vi "Main.vi"() -> ()   [LabVIEW 2012]
uses:
  <vilib>/addons/_XControls/Orbit Plot/SVX Orbit.xctl
  <vilib>/Math Plots/3D Math Plots/3D Surface/3D Surface XCtrl/3D Surface.xctl
  <vilib>/Utility/error.llb/DialogType.ctl
  <vilib>/Analysis/3filter.llb/Filter Passband Type.ctl
  <vilib>/DAQmx/read.llb/DAQmx Read (Analog 1D Wfm NChan NSamp).vi
  <vilib>/DAQmx/create/channels.llb/DAQmx Create Channel (AI-Position-EddyCurrentProxProbe).vi
  <vilib>/DAQmx/configure/timing.llb/DAQmx Timing (Sample Clock).vi
  <vilib>/Waveform/WDTOps.llb/WDT Append Waveforms DBL.vi
  <vilib>/Waveform/WDTOps.llb/WDT Index Channel DBL.vi
  <vilib>/Analysis/baseanly.llb/Mean (DBL).vi
  <vilib>/Waveform/WDTOps.llb/WDT Index Channel by Name DBL.vi
  <vilib>/Analysis/3filter.llb/Butterworth Filter (DBL).vi
  <vilib>/DAQmx/miscellaneous.llb/DAQmx Fill In Error Info.vi
  <resource>/objmgr/daqmx.rc
  <vilib>/Analysis/NI_AALBase.lvlib
  <vilib>/addons/Sound and Vibration/Order Analysis/Tach Process/SoundVib_TachProcess.lvlib
panel:
  out "3D Surface":refnum<class "3D Plot Datatype.lvclass">[](xcontrol)
  out "owmax":dbl
  out "Oil Whirl":T1(graph)
  out "Freq [Hz]":dbl
  out "deltaphase":dbl
  out "even-angle references":cluster{"r0":dbl, "dr":dbl, "Y":dbl[]}[](array[cluster])
  out "Magcri2":dbl
  out "Freq [Hz]":dbl
  out "Partial Rub":T1(graph)
  out "Freq [Hz]":dbl
  out "MATSCRIPT error 3":errorcluster
  out "prmax":dbl
  out "FreqFspec":T2(array[cluster])
  out "Freq [Hz]":dbl
  out "Unbalance":T1(graph)
  out "Freq crit":dbl
  out "Magcrit":dbl
  out "Radial Load/ Rotor cracked":T1(graph)
  out "RotMagdeltaphase":dbl[](array[numeric])
  out "MATSCRIPT error 2":errorcluster
  out "Full Spectro error":errorcluster
  out "error dequeue 2":errorcluster caption="error out"
  out "# elements in queue FS":i32
  out "> Limit":bool
  out "Actual Sample Rate (dt)":dbl
  out "MATSCRIPT error":errorcluster
  out "RPMs Calculados":i32
  out "Channels and Names":string[][](array[string])
  in  "Start":bool
  out "State":T3(ring)
  out "error dequeue":errorcluster caption="error out"
  out "Mag/F":errorcluster
  out "no tacho?":bool
  out "# elements in queue":i32
  out "> limit":bool
  in  "Stop":bool
  in  "Tab Control":T4(tab)
  in  "Names":string[](array[string])
  in  "Min Sample Rate [Hz]":dbl=10000.0
  in  "Maximum Value":dbl=0.0025 format="%.5f"
  in  "Units":i32(ring)=10219 items=["Meters"=10219, "Inches"=10379, "From Custom Scale"=10065]
  in  "Sensitivity":dbl=7.87
  in  "Sensitivity Units":i32(ring)=14839 items=["mVolts/mil"=14836, "Volts/mil"=14837, "mVolts/mm"=14838, "Volts/mm"=14839, "mVolts/micron"=14840]
  in  "Minimum Value":dbl=0.0002 format="%.5f"
  in  "DAQmx Selector":cluster{"On":bool, "physical channels":tag}[](array[cluster])=[{"On"=TRUE, "physical channels"="cDAQ2Mod1/ai0"}, {"On"=TRUE, "physical channels"="cDAQ2Mod1/ai1"}, {"On"=TRUE, "physical channels"="cDAQ2Mod1/ai2"}, {"On"=TRUE, "physical channels"="cDAQ2Mod2/ai0"}]
  in  "Keyphasor":tag="cDAQ2Mod2/ai1"
  in  "Threshold":dbl=0.0001
  in  "Direction":enum16{"CCW", "CW"}(ring)
  out "Actual Sample Rate [Hz]":dbl
  in  "Probe Angle X [deg]":u16
  in  "Probe Angle Y [deg]":u16=90
  out "Keyphasor":waveform(dbl)(graph)
  out "Radial Sensors":waveform(dbl)[](graph)
  in  "Write to File?":bool
  in  "TDMS File Path":path=path "C:/Users/Clayton/Documents/Mestrado ITA/Dissertacao/Simulacoes Matlab/zLabView/TDMS_teste.tdms"
  in  "Axis Y - Orbit 2":i8(ring) items=["x1", "y1", "x2", "y2"]
  in  "Axis X - Orbit 1":i8(ring) items=["x1", "y1", "x2", "y2"]
  out "Orbit 1":cluster{"Y":dbl[], "Y":dbl[]}(graph)
  out "Orbit 2":cluster{"Y":dbl[], "Y":dbl[]}(graph)
  in  "Axis Y - Orbit 1":i8(ring) items=["x1", "y1", "x2", "y2"]
  in  "Axis X - Orbit 2":i8(ring) items=["x1", "y1", "x2", "y2"]
  in  "Automatic":dbl=10.0
  in  "Duration [Rotation]":dbl=10.0 format="%.2f"
  in  "Sensor Y":i8(ring) items=["x1", "y1", "x2", "y2"]
  in  "Sensor X":i8(ring) items=["x1", "y1", "x2", "y2"]
  out "Full Spectrum":T1(graph)
  in  "Window":u32(ring)=1 items=["None"=0, "Hanning"=1, "Hamming"=2, "Blackman-Harris"=3, "Exact Blackman"=4, "Blackman"=5, "Flat Top"=6, "4 Term B-Harris"=7, "7 Term B-Harris"=8, "Low Sidelobe"=9, "Gaussian"=62]
  out "Rotor Crack":dbl(slide) scale=0.0..1.0
  out "Partial Rub":dbl(slide) scale=0.0..1.0
  out "Radial Load":dbl(slide) scale=0.0..1.0
  out "Unbalance":dbl(slide) scale=0.0..1.0
  out "Oil Whirl":dbl(slide) scale=0.0..1.0
  out "Rotation [rps]":dbl format="%#.4f"
  out "Error Matlab Script":bool
  out "Error Full Spectrum":bool
  in  "Compensate":bool
  in  "Reset":bool
  out "Orbit Plot":T5(xcontrol)
  in  "Freq. Diagnosis [rps]":dbl=50.0
  in  "Simulation path":path=path "C:/Users/Clayton/Documents/Mestrado ITA/Dissertacao/Simulacoes Matlab/zLabView/TDMS_teste.tdms"
  in  "Simulation":bool
  in  "Sensor X":i32=1
  in  "Sensor Y":i32=2
  out "Phase":cluster{dbl[], dbl[]}(graph)
  in  "Order":i8(ring) items=["1x", "2x"]
  out "Magnitude":cluster{dbl[], dbl[]}(graph)
  out "Phase":cluster{dbl[], dbl[]}(graph)
  out "Magnitude":cluster{dbl[], dbl[]}(graph)
  in  "Order":i8(ring) items=["1x", "2x"]
  out "Sensor":string
  out "Sensor":string
  # "Slow Roll"
  # "Diagnosis"
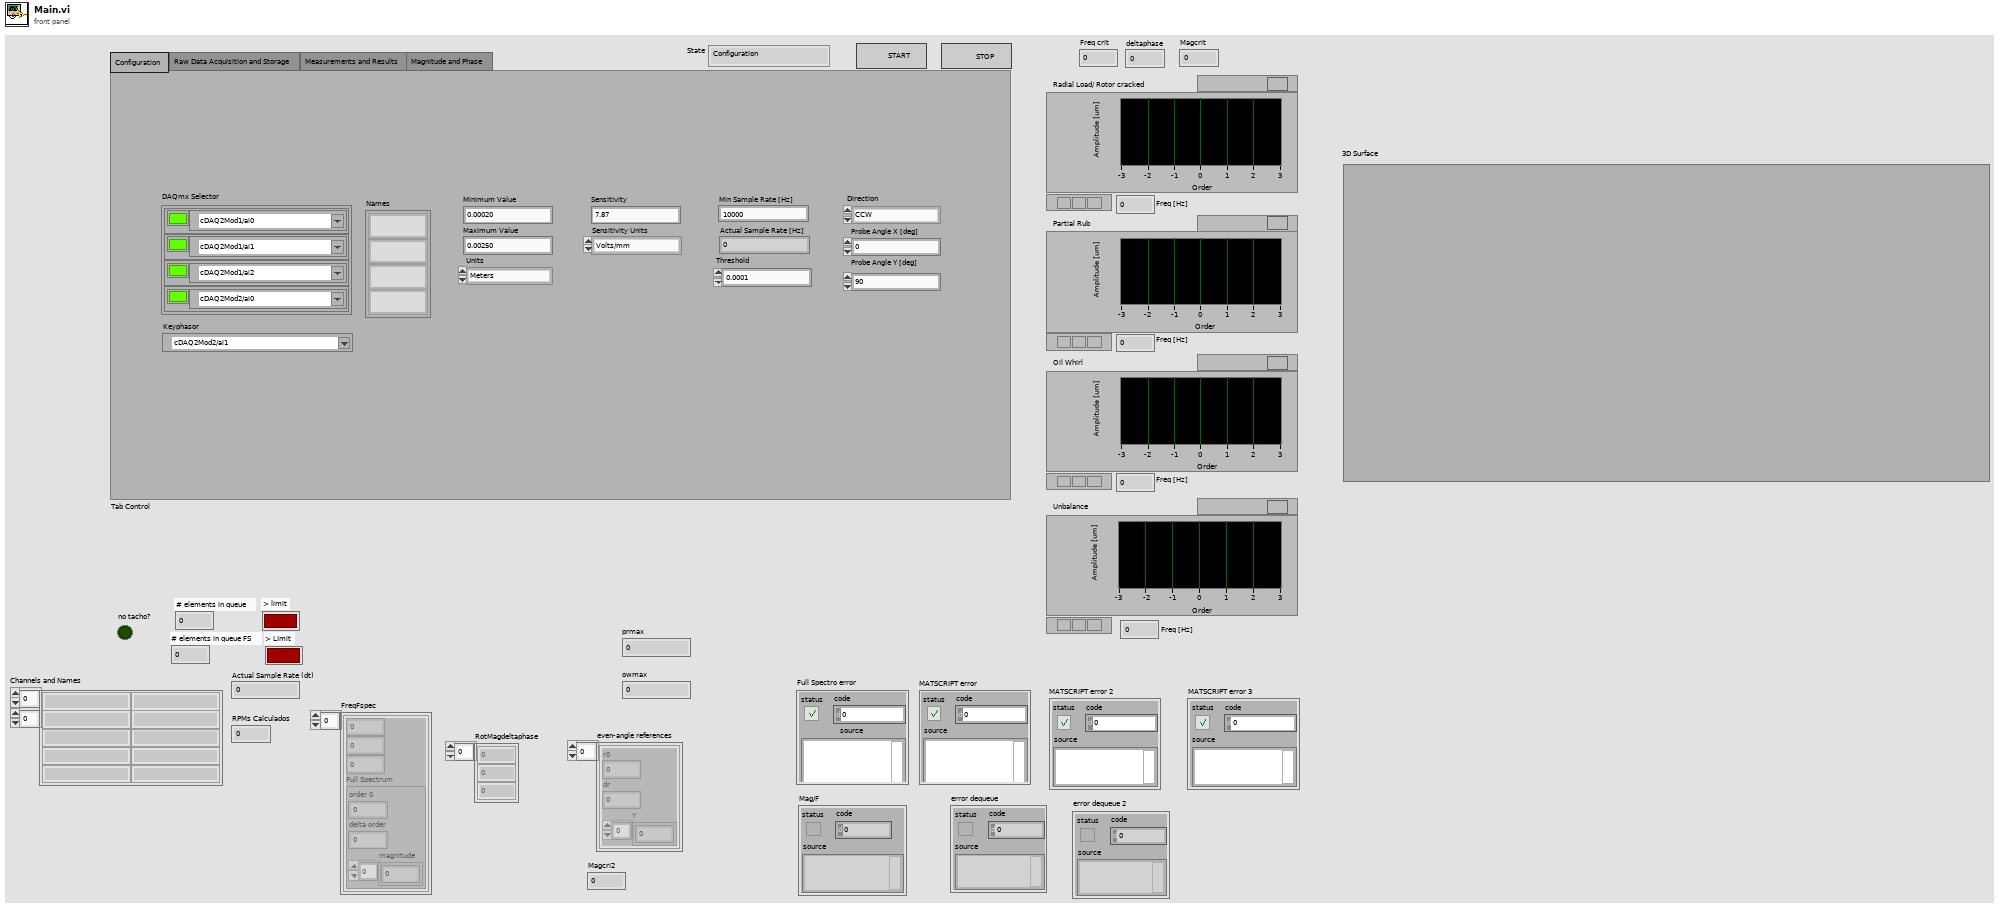
[diagram p1: front panel]
types:
  T1 = cluster{"order 0":dbl, "delta order":dbl, "magnitude":dbl[]}
  T2 = cluster{dbl, dbl, dbl, "Full Spectrum":cluster{"order 0":dbl, "delta order":dbl, "magnitude":dbl[]}}[]
  T3 = enum16{"Configuration", "Initializing", "RUNNING"}
  T4 = enum32{"Configuration", "Raw Data Acquisition and Storage", "Measurements and Results", "Magnitude and Phase"}
  T5 = cluster{"probe x":dbl[], "probe y":dbl[], "reference":dbl[], "plot type":enum16{"Filtered Plot", "Unfiltered Plot"}, "attribute":variant}[][]
  T6 = enum8{"Enabled", "Disabled", "Disabled and Grayed Out"}
  T7 = enum16{"open", "open or create", "create or replace", "create", "open (read-only)"}
  T8 = cluster{"dB on? (F)":bool, "unwrap phase? (T)":bool, "unit in degree? (T)":bool}
  T9 = typedef "DialogType.ctl" = u16
  T10 = typedef "NI_AALBase.lvlib/Filter Passband Type.ctl" = enum32{"Lowpass", "Highpass", "Bandpass", "Bandstop"}
  T11 = cluster{dbl, dbl, dbl, "Full Spectrum":cluster{"order 0":dbl, "delta order":dbl, "magnitude":dbl[]}}
  T12 = typedef "SoundVib_TachProcess.lvlib/speed profile.ctl" = cluster{"time [s]":dbl[], "speed [RPM]":dbl[]}
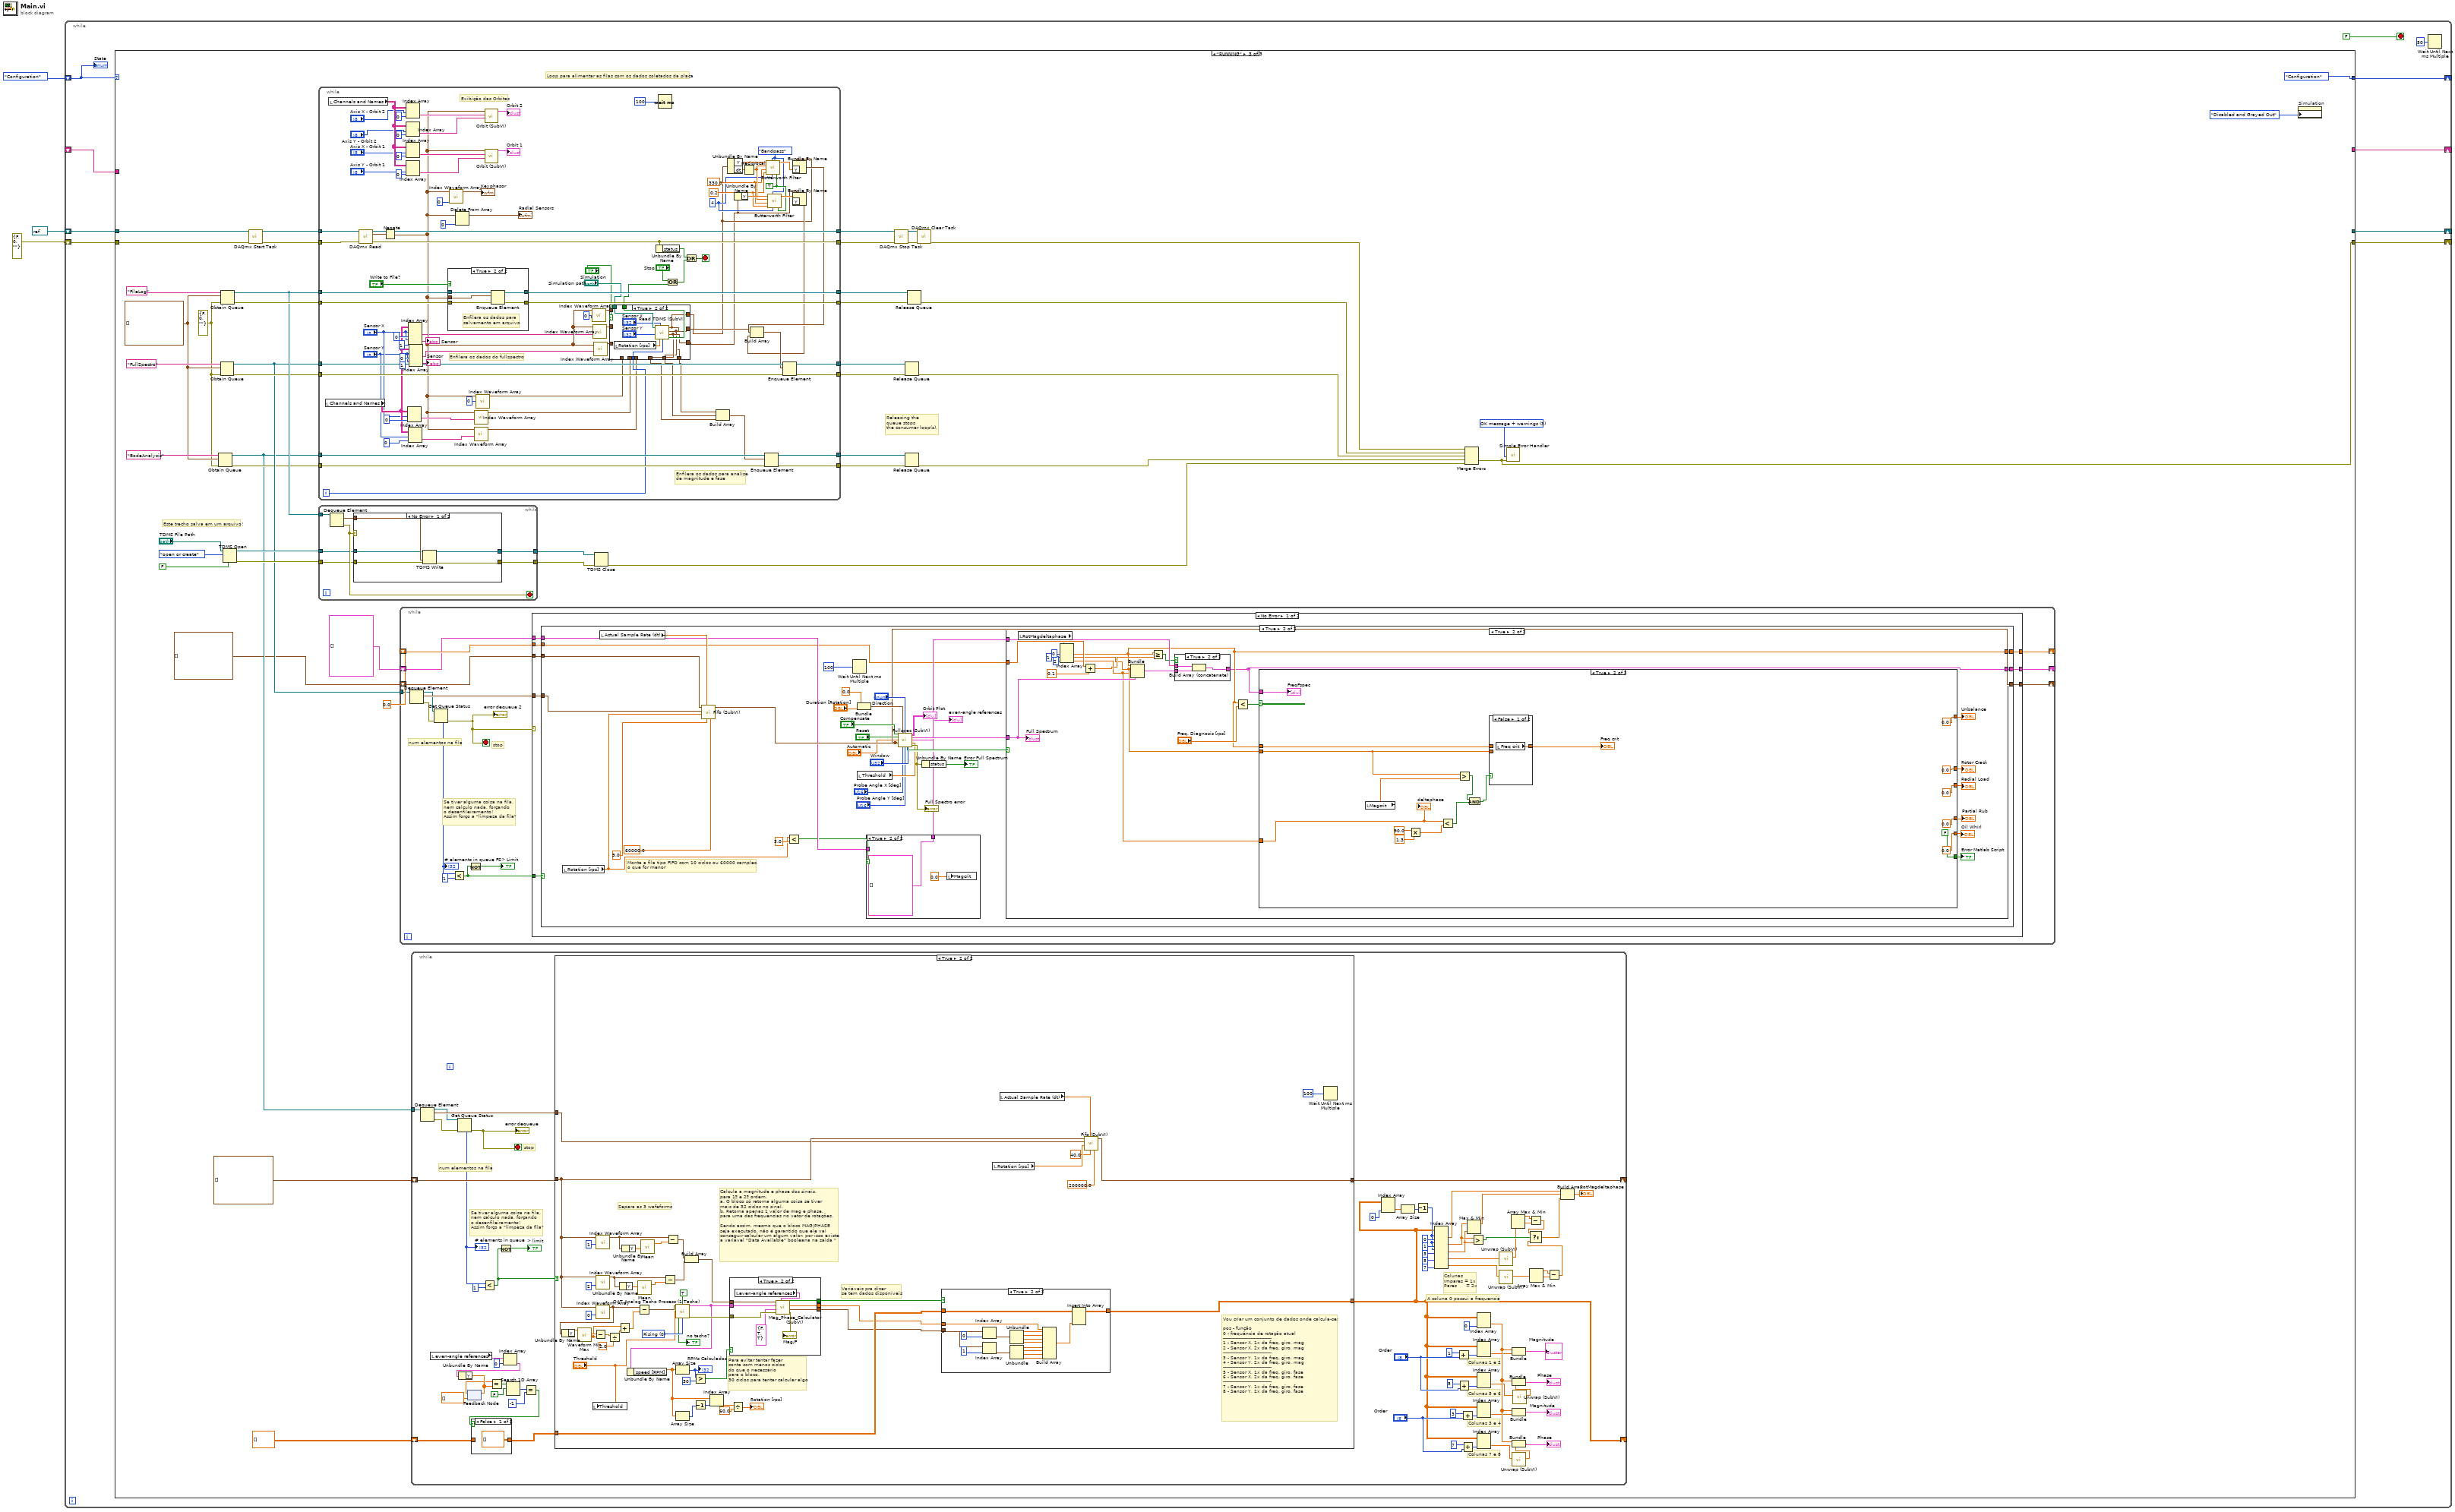
[diagram p0: block diagram]
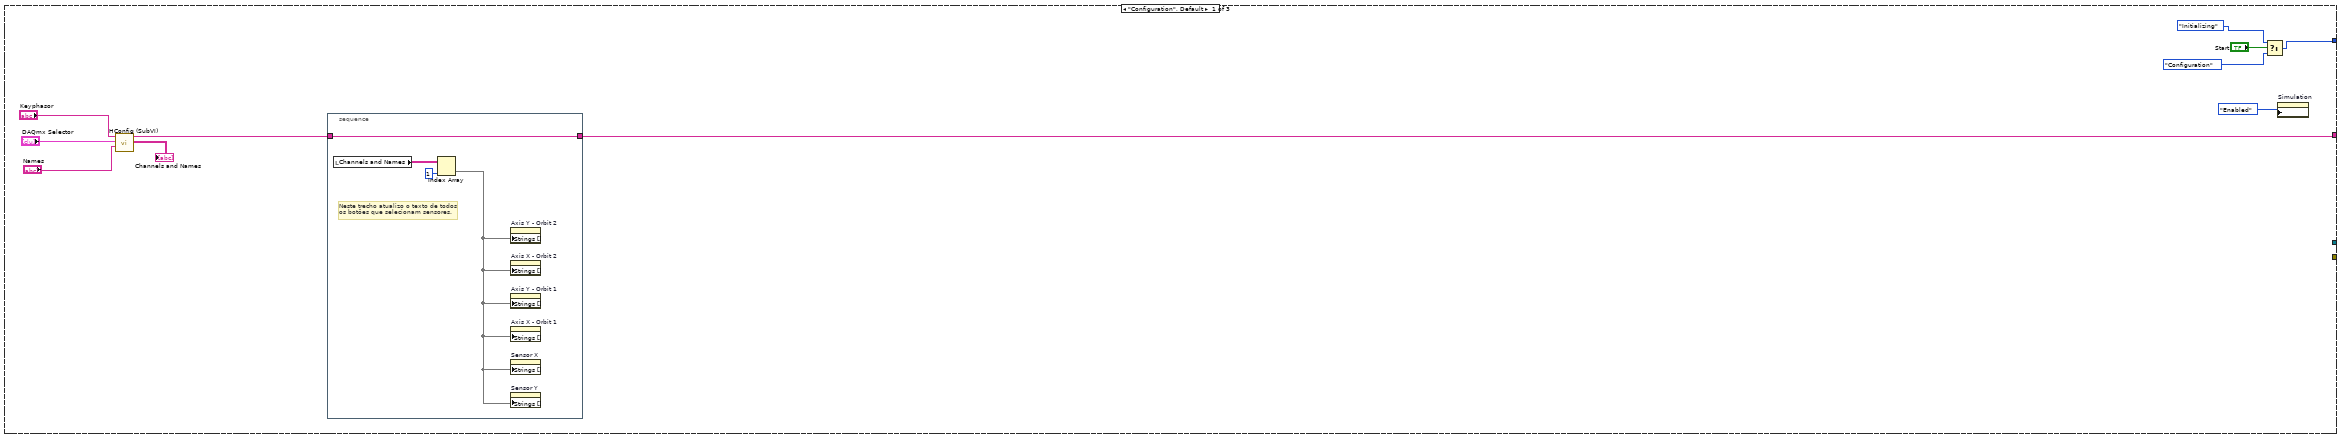
[diagram p2: hidden frame]
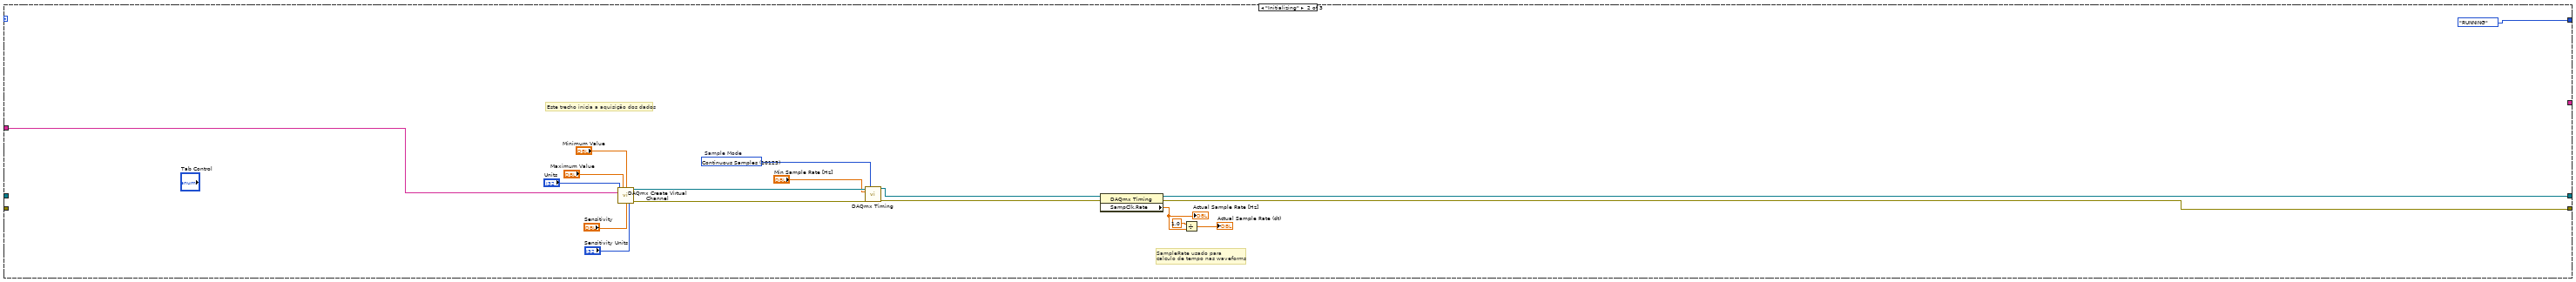
[diagram p3: hidden frame]
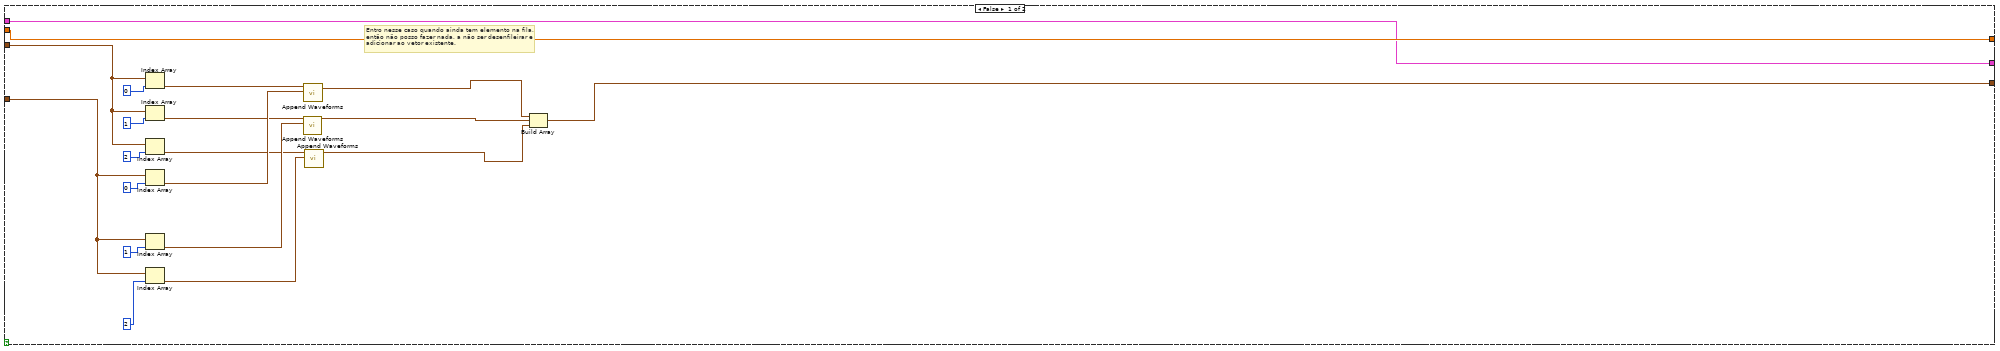
[diagram p4: hidden frame]
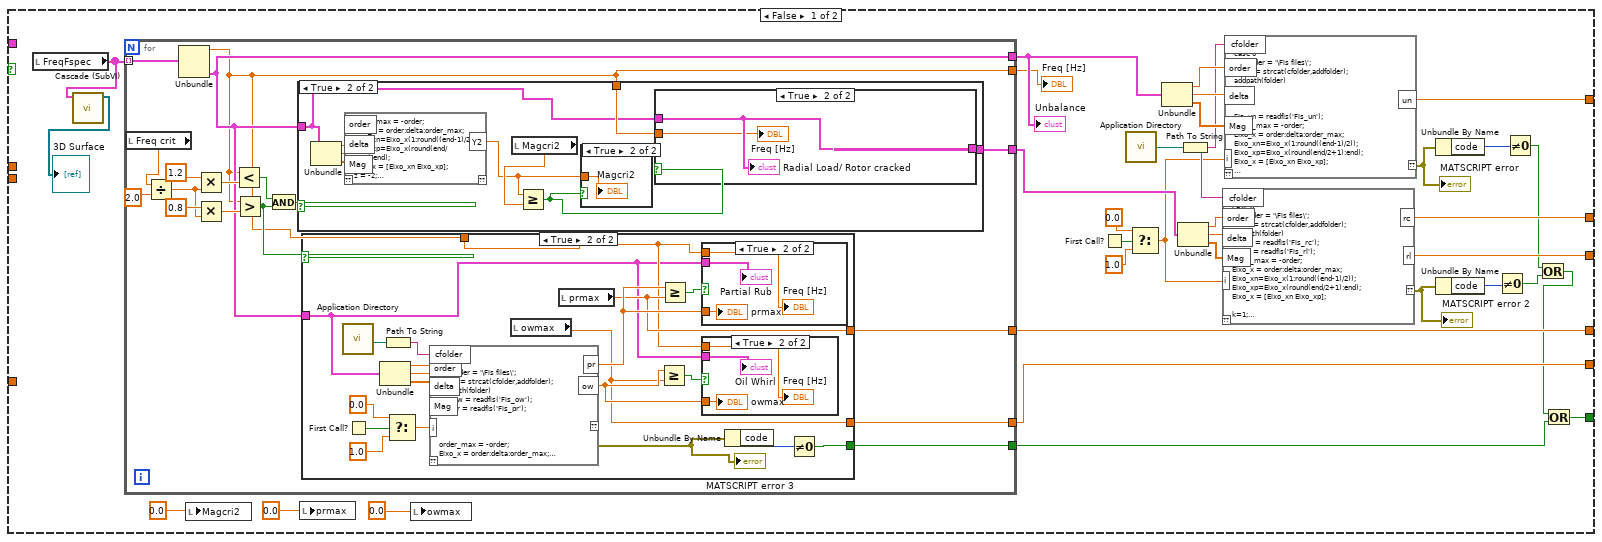
[diagram p7: hidden frame]
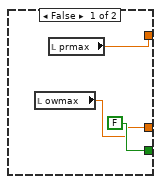
[diagram p8: hidden frame]
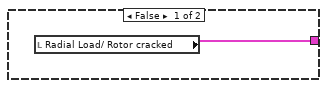
[diagram p11: hidden frame]
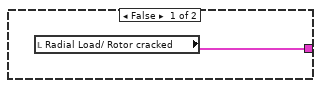
[diagram p13: hidden frame]
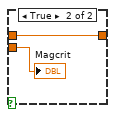
[diagram p14: hidden frame]
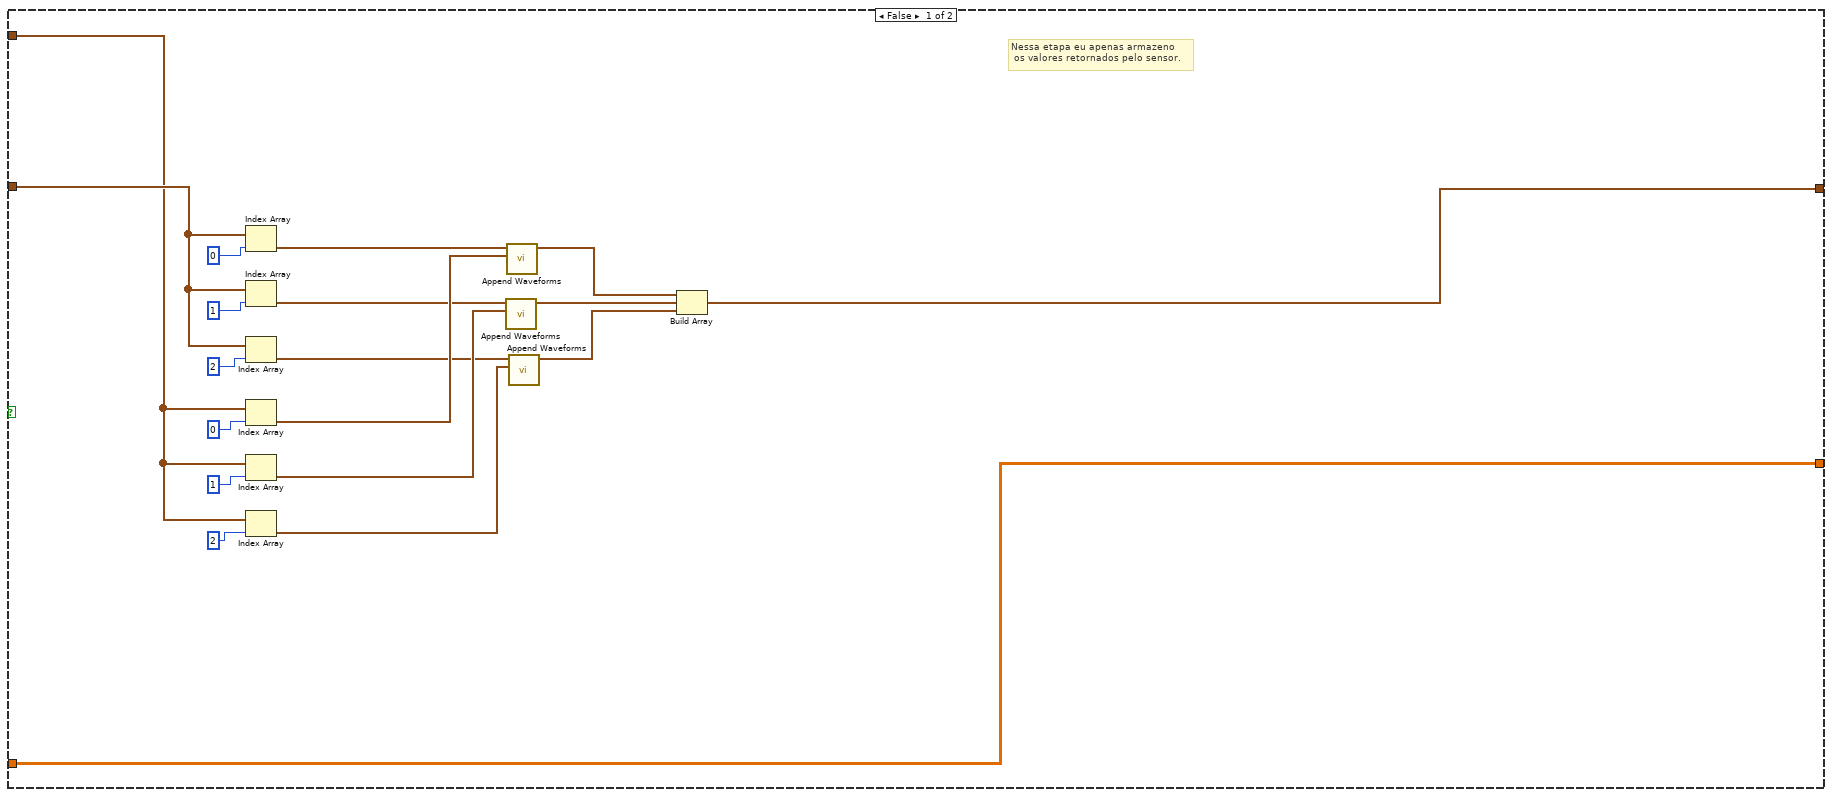
[diagram p18: hidden frame]
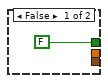
[diagram p20: hidden frame]
diagram:
  n1 = while {
    shift-right: [w4] -> _
    shift-left: T3."Configuration" ("Enum") -> [w9]
    shift-right: [w13] -> _
    shift-left: refnum<k21> refnum ("task out") -> [w12]
    shift-right: [w10] -> _
    shift-left: errorcluster {"status"=FALSE, "code"=0, "source"=""} ("error in (no error)") -> [w11]
    shift-right: [w8] -> _
    shift-left: _ -> [w7]
    stop <- FALSE stop-if-true
    n2 = case shown="\"RUNNING\"" w9 {
      tunnel: [_ w34 _] -> w13
      tunnel: [_ w33 w62] -> w10
      tunnel: w12 -> [_ _ w59]
      tunnel: w11 -> [_ _ w58]
      tunnel: [w19 T3."RUNNING" ("Enum") T3."Configuration" ("Enum")] -> w4
      tunnel: [w17 _ _] -> w8
      tunnel: w7 -> [_ w30 _]
      frame "Configuration", Default {
        n3 = call "HConfig (SubVI).vi"("Names"="Names", "DAQmx Selector"="DAQmx Selector", "Keyphasor"="Keyphasor") -> ("Channels and Names"=→"Channels and Names":string[][], "String"=w18:string)  [unwired: 7 in]
        n4 = stacked-sequence {
          tunnel: w18 -> [w25]
          tunnel: [w25] -> w17
          frame #0 {
            # "Neste trecho atualizo o texto de todos \nos botões que selecionam sensores."
            n5 = local read "Channels and Names"() -> (w28:string[][])
            n6 = Index Array(array=w28, index (col)=1 ("disabled index (col)")) -> (element=w26:string[])  [unwired: 1 in]
            n7 = property on="Axis Y - Orbit 2" class="Ring (strict)"("Strings []"=w26) -> ()  [unwired: 2 in, 2 out]
            n8 = property on="Axis X - Orbit 2" class="Ring (strict)"("Strings []"=w26) -> ()  [unwired: 2 in, 2 out]
            n9 = property on="Axis Y - Orbit 1" class="Ring (strict)"("Strings []"=w26) -> ()  [unwired: 2 in, 2 out]
            n10 = property on="Axis X - Orbit 1" class="Ring (strict)"("Strings []"=w26) -> ()  [unwired: 2 in, 2 out]
            n11 = property on="Sensor X" class="Ring (strict)"("Strings []"=w26) -> ()  [unwired: 2 in, 2 out]
            n12 = property on="Sensor Y" class="Ring (strict)"("Strings []"=w26) -> ()  [unwired: 2 in, 2 out]
          }
        }
        n13 = Select(t=T3."Initializing" ("Enum"), s="Start", f=T3."Configuration" ("Enum")) -> (s? t:f=w19:T3)
        n14 = property on="Simulation" class="Bool (strict)"("DisabledEnum"=T6."Enabled" ("Disabled")) -> ()  [unwired: 2 in, 2 out]
      }
      frame "Initializing" {
        w35 = 10123 items=["Finite Samples"=10178, "Continuous Samples"=10123, "Hardware Timed Single Point"=12522]  # Sample Mode
        # "SampleRate usado para \ncalculo de tempo nas waveforms"
        # "Este trecho inicia a aquisição dos dados"
        n15 = call-poly <vilib>:"DAQmx Create Virtual Channel.vi"("maximum value"="Maximum Value", "minimum value"="Minimum Value", "physical channels"=w30, "units"="Units", "sensitivity"="Sensitivity", "sensitivity units"="Sensitivity Units") -> ("task out"=w42:refnum<k21>, "error out"=w43:errorcluster)  [unwired: 8 in]
        n16 = call-poly <vilib>:"DAQmx Timing.vi"("task/channels in"=w42, "sample mode"=w35, "rate"="Min Sample Rate [Hz]", "error in"=w43) -> ("task out"=w44:refnum<k21>, "error out"=w45:errorcluster)  [unwired: 10 in]
        n17 = property class="DAQmx Timing"(reference=w44, error in=w45) -> (reference out=w34:refnum<k21>, error out=w33:errorcluster, "SampClk.Rate"=w29:dbl)
        "Actual Sample Rate [Hz]" <- w29
        n18 = Divide(x=1.0, y=w29) -> (x/y=→"Actual Sample Rate (dt)":dbl)
      }
      frame "RUNNING" {
        w54 = waveform(dbl)[] [] ("Measurement 2")
        w53 = errorcluster {"status"=FALSE, "code"=0, "source"=""} ("error in (no error)")
        w88 = T9 3 items=["no dialog", "OK message", "continue or stop message", "OK message + warnings", "continue/stop + warnings"] ("type of dialog (OK msg:1)")
        # "Este trecho salva em um arquivo!"
        # "Releasing the\nqueue stops\nthe consumer loop(s)."
        # "Loop para alimentar as filas com os dados coletados da placa"
        n19 = Obtain Queue(name (unnamed)="BodeAnalysis", element data type=w54, error in (no error)=w53) -> (queue out=w65:refnum<queue>, error out=w71:errorcluster)  [unwired: 2 in, 1 out]
        n20 = Obtain Queue(name (unnamed)="FullSpectro", element data type=w54, error in (no error)=w53) -> (queue out=w75:refnum<queue>, error out=w76:errorcluster)  [unwired: 2 in, 1 out]
        n21 = Obtain Queue(name (unnamed)="FileLog", element data type=w54, error in (no error)=w53) -> (queue out=w80:refnum<queue>, error out=w87:errorcluster)  [unwired: 2 in, 1 out]
        n22 = TDMS Open(6:FALSE ("disable buffering (T)"), 10:T7."open or create" ("operation"), 11:"TDMS File Path") -> (0:w82:errorcluster, 3:w83:refnum<k34>)  [unwired: 3 in]
        n23 = call <vilib>:"DAQmx Start Task.vi"("task/channels in"=w59, "error in"=w58) -> ("task out"=w61:refnum<k21>, "error out"=w60:errorcluster)  [unwired: 12 in]
        n24 = while {
          tunnel: w61 -> [w590]
          tunnel: w60 -> [w589]
          tunnel: [w593] -> w92
          tunnel: [w583] -> w91
          tunnel: w80 -> [w587]
          tunnel: w87 -> [w586]
          tunnel: [w585] -> w86
          tunnel: [w584] -> w79
          tunnel: w75 -> [w577]
          tunnel: [w576] -> w78
          tunnel: [w575] -> w77
          tunnel: w76 -> [w574]
          tunnel: [w572] -> w74
          tunnel: w65 -> [w573]
          tunnel: [w571] -> w72
          tunnel: w71 -> [w570]
          i -> [w510]
          stop <- w591 stop-if-true
          w530 = TRUE ("init/cont (init:F)")
          w532 = 0.2 ("low cutoff freq: fl")
          w533 = 330.0 ("high cutoff freq: fh")
          w531 = 4 ("order")
          w529 = Filter_Passband_Type."Bandpass" ("filter type")
          # "Enfilera os dados do fullspectro"
          # "Enfilera os dados para análise \nde magnitude e fase"
          # "Exibição das Orbitas"
          n25 = local read "Channels and Names"() -> (w547:string[][])
          n26 = local read "Channels and Names"() -> (w559:string[][])
          n27 = call-poly <vilib>:"DAQmx Read.vi"("task/channels in"=w590, "error in"=w589) -> ("task out"=w593:refnum<k21>, "data"=w543:waveform(dbl)[], "error out"=w583:errorcluster)  [unwired: 11 in]
          n28 = Negate(x=w543) -> (-x=w544:waveform(dbl)[])
          n29 = Index Array(array=w559, index (row)="Axis X - Orbit 2", index (col)=0) -> (element=w551:string)
          n30 = Index Array(array=w559, index (row)="Axis Y - Orbit 2", index (col)=0) -> (element=w552:string)
          n31 = Index Array(array=w559, index (row)="Axis X - Orbit 1", index (col)=0) -> (element=w555:string)
          n32 = Index Array(array=w559, index (row)="Axis Y - Orbit 1", index (col)=0) -> (element=w557:string)
          n33 = Index Array(array=w547, index (row)="Sensor X", index (col)=0 ("disabled index (col)")) -> (element=w566:string)
          n34 = Index Array(array=w547, index (row)="Sensor Y", index (col)=0 ("disabled index (col)")) -> (element=w564:string)
          n35 = Index Array(array=w547, index (row) #1="Sensor X", index (col) #1=0 ("index (col)"), index (row) #2="Sensor X", index (col) #2=1 ("index (col)")) -> (element #1=w520:string, element #2=→"Sensor":string)
          n36 = Index Array(array=w547, index (row) #1="Sensor Y", index (col) #1=0 ("index (col)"), index (row) #2="Sensor Y", index (col) #2=1 ("disabled index (col)")) -> (element #1=w519:string, element #2=→"Sensor":string)
          n37 = case shown="True" "Write to File?" {
            tunnel: [w611 w616] -> w585
            tunnel: [w610 w615] -> w584
            tunnel: w587 -> [w611 w614]
            tunnel: w586 -> [w610 w613]
            tunnel: w544 -> [_ w612]
            frame False {
            }
            frame True {
              # "Enfilera os dados para \nsalvamento em arquivo"
              n38 = Enqueue Element(queue=w614, element=w612, error in (no error)=w613) -> (queue out=w616:refnum<queue>, error out=w615:errorcluster)  [unwired: 2 out]
            }
          }
          n39 = call-poly <vilib>:"Index Waveform Array.vi"("index"=0, "waveform array"=w544) -> ("waveform"=→"Keyphasor":waveform(dbl))  [unwired: 8 in, 1 out]
          n40 = Delete From Array(array=w544, index=0) -> (array with subset deleted=→"Radial Sensors":waveform(dbl)[])  [unwired: 1 in, 1 out]
          n41 = call-poly <vilib>:"Index Waveform Array.vi"("channel name"=w564, "waveform array"=w544) -> ("waveform"=w504:waveform(dbl))  [unwired: 8 in, 1 out]
          n42 = call-poly <vilib>:"Index Waveform Array.vi"("channel name"=w566, "waveform array"=w544) -> ("waveform"=w505:waveform(dbl))  [unwired: 8 in, 1 out]
          n43 = call-poly <vilib>:"Index Waveform Array.vi"("index"=0, "waveform array"=w544) -> ("waveform"=w506:waveform(dbl))  [unwired: 8 in, 1 out]
          n44 = call "Orbit (SubVI).vi"("Axis Y1"=w552, "Axis X1"=w551, "Array"=w544) -> ("Cluster"=→"Orbit 2":cluster{"Y":dbl[], "Y":dbl[]})  [unwired: 7 in, 1 out]
          n45 = call "Orbit (SubVI).vi"("Axis Y1"=w557, "Axis X1"=w555, "Array"=w544) -> ("Cluster"=→"Orbit 1":cluster{"Y":dbl[], "Y":dbl[]})  [unwired: 7 in, 1 out]
          n46 = call-poly <vilib>:"Index Waveform Array.vi"("index"=0, "waveform array"=w544) -> ("waveform"=w509:waveform(dbl))  [unwired: 8 in, 1 out]
          n47 = call-poly <vilib>:"Index Waveform Array.vi"("channel name"=w520, "waveform array"=w544) -> ("waveform"=w508:waveform(dbl))  [unwired: 8 in, 1 out]
          n48 = call-poly <vilib>:"Index Waveform Array.vi"("channel name"=w519, "waveform array"=w544) -> ("waveform"=w507:waveform(dbl))  [unwired: 8 in, 1 out]
          n49 = case shown="True" "Simulation" {
            tunnel: "Simulation path" -> [_ w608]
            tunnel: [FALSE ("stop") w607] -> w512
            tunnel: w510 -> [_ w606]
            tunnel: [w600 w603] -> w518
            tunnel: [w599 w604] -> w517
            tunnel: [w598 w605] -> w516
            tunnel: [w597 w605] -> w513
            tunnel: [w596 w604] -> w514
            tunnel: [w595 w603] -> w515
            tunnel: w509 -> [w600 _]
            tunnel: w508 -> [w599 _]
            tunnel: w507 -> [w598 _]
            tunnel: w504 -> [w597 _]
            tunnel: w505 -> [w596 _]
            tunnel: w506 -> [w595 _]
            frame False {
            }
            frame True {
              n50 = local read "Rotation [rps]"() -> (w609:dbl)
              n51 = call "Read TDMS (SubVI).vi"("Sensor Y"="Sensor Y", "Sensor X"="Sensor X", "Rotation"=w609, "i"=w606, "TDMS File Path in"=w608) -> ("stop"=w607:bool, "waveform 3"=w605:waveform(dbl), "waveform 2"=w604:waveform(dbl), "waveform 1"=w603:waveform(dbl))  [unwired: 3 in]
            }
          }
          n52 = Unbundle By Name(w583) -> ("status"=w592:bool)
          n53 = Wait (ms)(milliseconds to wait=u32 100) -> ()  [unwired: 1 out]
          n54 = Or(x="Stop", y=w512) -> (x .or. y?=w522:bool)
          n55 = Or(x=w592, y=w522) -> (x .or. y?=w591:bool)
          n56 = Build Array(w515, w514, w513) -> (w568:waveform(dbl)[])
          n57 = Unbundle By Name(w517) -> ("Y"=w541:dbl[], "dt"=w540:dbl)
          n58 = Unbundle By Name(w516) -> ("Y"=w537:dbl[])
          n59 = Reciprocal(x=w540) -> (1/x=w534:dbl)
          n60 = Enqueue Element(queue=w573, element=w568, error in (no error)=w570) -> (queue out=w572:refnum<queue>, error out=w571:errorcluster)  [unwired: 1 in, 1 out]
          n61 = call-poly <vilib>:"Butterworth Filter.vi"("init/cont (init:F)"=w530, "order"=w531, "filter type"=w529, "low cutoff freq: fl"=w532, "high cutoff freq: fh"=w533, "sampling freq: fs"=w534, "X"=w541) -> ("Filtered X"=w539:dbl[])  [unwired: 1 in, 1 out]
          n62 = call-poly <vilib>:"Butterworth Filter.vi"("init/cont (init:F)"=w530, "order"=w531, "filter type"=w529, "low cutoff freq: fl"=w532, "high cutoff freq: fh"=w533, "sampling freq: fs"=w534, "X"=w537) -> ("Filtered X"=w536:dbl[])  [unwired: 1 in, 1 out]
          n63 = Bundle By Name(cluster=w517, "Y"=w539) -> (w538:waveform(dbl))
          n64 = Bundle By Name(cluster=w516, "Y"=w536) -> (w535:waveform(dbl))
          n65 = Build Array(w518, w538, w535) -> (w542:waveform(dbl)[])
          n66 = Enqueue Element(queue=w577, element=w542, error in (no error)=w574) -> (queue out=w576:refnum<queue>, error out=w575:errorcluster)  [unwired: 2 out]
        }
        n67 = while {
          tunnel: w80 -> [w495]
          tunnel: [w492] -> w56
          tunnel: [w491] -> w55
          tunnel: w83 -> [w490]
          tunnel: w82 -> [w489]
          stop <- w494 stop-if-true
          n68 = Dequeue Element(queue=w495) -> (element=w493:waveform(dbl)[], error out=w494:errorcluster)  [unwired: 1 in, 3 out]
          n69 = case shown="No Error" w494 {
            tunnel: w493 -> [w498 _]
            tunnel: [w499 w502] -> w492
            tunnel: [w500 w501] -> w491
            tunnel: w490 -> [w497 w502]
            tunnel: w489 -> [w496 w501]
            frame No Error {
              n70 = TDMS Write(0:w497, 9:w498, 11:w496) -> (4:w499:refnum<k34>, 15:w500:errorcluster)  [unwired: 3 in, 2 out]
            }
            frame Error {
            }
          }
        }
        n71 = while {
          tunnel: w75 -> [w107]
          shift-right: [w99] -> _
          shift-left: waveform(dbl)[] [] ("appended array") -> [w100]
          shift-right: [w93] -> _
          shift-left: 0.0 -> [w96]
          shift-right: [w95] -> _
          shift-left: T2 [] -> [w94]
          stop <- w98 stop-if-true
          # "num elementos na fila"
          # "Se tiver alguma coisa na fila,\nnem calculo nada, forçando \no desenfileiramento!\nAssim forço a \"limpeza da fila\""
          # "stop"
          n72 = Dequeue Element(queue=w107) -> (queue out=w102:refnum<queue>, element=w106:waveform(dbl)[], error out=w101:errorcluster)  [unwired: 1 in, 2 out]
          n73 = Get Queue Status(queue=w102, error in (no error)=w101) -> (error out=w98:errorcluster, # elements in queue=w105:i32)  [unwired: 1 in, 6 out]
          "error dequeue 2" <- w98
          "# elements in queue FS" <- w105
          n74 = Less?(x=w105, y=1) -> (x < y?=w97:bool)
          n75 = Not(x=w97) -> (.not. x?=→"> Limit":bool)
          n76 = case shown="No Error" w98 {
            tunnel: w106 -> [w115 _]
            tunnel: w100 -> [w114 w317]
            tunnel: [w113 w317] -> w99
            tunnel: w97 -> [w112 _]
            tunnel: [w111 w316] -> w93
            tunnel: w96 -> [w110 w316]
            tunnel: [w109 w315] -> w95
            tunnel: w94 -> [w108 w315]
            frame No Error {
              n77 = case shown="True" w112 {
                tunnel: w115 -> [w123 w162]
                tunnel: w114 -> [w122 w160]
                tunnel: [w121 w151] -> w113
                tunnel: [w117 w145] -> w111
                tunnel: w110 -> [w117 w139]
                tunnel: [w116 w144] -> w109
                tunnel: w108 -> [w116 w143]
                frame False {
                  # "Entro nesse caso quando ainda tem elemento na fila, \nentão não posso fazer nada, a não ser desenfileirar e \nadicionar ao vetor existente."
                  n78 = Index Array(array=w122, index=0 ("disabled index (col)")) -> (element=w129:waveform(dbl))
                  n79 = Index Array(array=w122, index=1 ("disabled index (col)")) -> (element=w127:waveform(dbl))
                  n80 = Index Array(array=w122, index=2 ("disabled index (col)")) -> (element=w125:waveform(dbl))
                  n81 = Index Array(array=w123, index=0 ("disabled index (col)")) -> (element=w128:waveform(dbl))
                  n82 = Index Array(array=w123, index=1 ("disabled index (col)")) -> (element=w126:waveform(dbl))
                  n83 = Index Array(array=w123, index=2 ("disabled index (col)")) -> (element=w124:waveform(dbl))
                  n84 = call-poly <vilib>:"Append Waveforms.vi"("waveform B"=w126, "waveform A"=w127) -> ("waveform out"=w119:waveform(dbl))  [unwired: 8 in, 1 out]
                  n85 = call-poly <vilib>:"Append Waveforms.vi"("waveform B"=w128, "waveform A"=w129) -> ("waveform out"=w120:waveform(dbl))  [unwired: 8 in, 1 out]
                  n86 = call-poly <vilib>:"Append Waveforms.vi"("waveform B"=w124, "waveform A"=w125) -> ("waveform out"=w118:waveform(dbl))  [unwired: 8 in, 1 out]
                  n87 = Build Array(w120, w119, w118) -> (w121:waveform(dbl)[])
                }
                frame True {
                  # "Monta a fila tipo FIFO com 10 ciclos ou 60000 samples, \no que for menor"
                  n88 = local read "Rotation [rps]"() -> (w138:dbl)
                  n89 = local read "Actual Sample Rate (dt)"() -> (w146:dbl)
                  n90 = call "Fifo (SubVI).vi"("duration"=60000.0, "y"=9.0, "Actual Sample Rate (dt)"=w146, "Rotation [RPS]"=w138, "Measurement in"=w162, "appended array"=w160) -> ("Array"=w151:waveform(dbl)[])  [unwired: 5 in]
                  n91 = Less?(x=w138, y=3.0) -> (x < y?=w141:bool)
                  n92 = Wait Until Next ms Multiple(millisecond multiple=u32 100 ("milliseconds to wait")) -> ()  [unwired: 1 out]
                  n93 = Bundle("start"=0.0, "Duration [Rotation]"="Duration [Rotation]") -> (w164:cluster{"start":dbl, "Duration [Rotation]":dbl})  [unwired: 1 in]
                  n94 = local read "Threshold"() -> (w155:dbl)
                  n95 = case shown="True" w141 {
                    tunnel: w143 -> [w168 _]
                    tunnel: [w168 T2 []] -> w142
                    frame False {
                    }
                    frame True {
                      n96 = local write "Magcrit"(0.0 ("Magcrit")) -> ()
                    }
                  }
                  n97 = call "Fullspec (SubVI).vi"("Compensate SR"="Compensate", "revolutions to display [rev]"=w164, "shaft rotating direction"="Direction", "Reset SR"="Reset", "AutSR"="Automatic", "Sensors"=w151, "threshold (auto)"=w155, "probe angle X [deg]"="Probe Angle X [deg]", "probe angle Y [deg]"="Probe Angle Y [deg]", "window"="Window") -> ("Execute  MATSCRIPT"=w158:bool, "orbit/timebase plot"=→"Orbit Plot":T5, "Full Spectrum"=w159:T1, "even-angle references"=→"even-angle references":cluster{"r0":dbl, "dr":dbl, "Y":dbl[]}[], "error out"=w157:errorcluster)  [unwired: 1 in]
                  "Full Spectro error" <- w157
                  n98 = Unbundle By Name(w157) -> ("status"=→"Error Full Spectrum":bool)
                  n99 = case shown="True" w158 {
                    tunnel: w159 -> [_ w185]
                    tunnel: [w171 w177] -> w145
                    tunnel: w139 -> [w171 w192]
                    tunnel: [w172 w175] -> w144
                    tunnel: w142 -> [w172 w194]
                    frame False {
                    }
                    frame True {
                      n100 = local read "RotMagdeltaphase"() -> (w189:dbl[])
                      n101 = Index Array(array=w189, index #1=0 ("index"), index #2=1 ("index"), index #3=2 ("index")) -> (element #1=w177:dbl, element #2=w176:dbl, element #3=w174:dbl)
                      n102 = Add(x=w192, y=0.1 ("Step [rps]")) -> (x+y=w191:dbl)
                      n103 = Bundle(w177, w176, w174, "Full Spectrum"=w185) -> (w193:T11)  [unwired: 1 in]
                      n104 = Greater Or Equal?(x=w177, y=w191) -> (x >= y?=w190:bool)
                      n105 = case shown="True" w190 {
                        tunnel: w193 -> [_ w312]
                        tunnel: [w311 w314] -> w175
                        tunnel: w194 -> [w311 w313]
                        frame False {
                        }
                        frame True {
                          n106 = Build Array (concatenate)(w313, w312) -> (w314:T2)
                        }
                      }
                      n107 = Less?(x=w177, y="Freq. Diagnosis [rps]") -> (x < y?=w186:bool)
                      n108 = case shown="True" w186 {
                        tunnel: w177 -> [_ w307]
                        tunnel: w175 -> [_ w298]
                        tunnel: w176 -> [_ w304]
                        tunnel: [w210 FALSE] -> w182
                        tunnel: [w209 0.0] -> w181
                        tunnel: [w208 0.0] -> w180
                        tunnel: [w207 0.0] -> w179
                        tunnel: [w203 0.0] -> w173
                        tunnel: [w202 0.0] -> w178
                        tunnel: w174 -> [_ w297]
                        frame False {
                          n109 = local read "FreqFspec"() -> (w199:T2)
                          n110 = call "Cascade (SubVI).vi"("FreqFspec in"=w199) -> ("3D Plot lvclass Array out"=→"3D Surface":refnum<class "3D Plot Datatype.lvclass">[])  [unwired: 10 in]
                          n111 = for {
                            tunnel: w199 -> [w246] mode=indexing
                            tunnel: [w245] -> w229
                            tunnel: [w234] -> w214
                            tunnel: [w233] -> w213
                            tunnel: [w232] -> w204
                            tunnel: [w231] -> w203
                            tunnel: [w230] -> w202
                            n112 = local read "Freq crit"() -> (w236:dbl)
                            n113 = Divide(x=w236, y=2.0) -> (x/y=w242:dbl)
                            n114 = Unbundle(w246) -> (w233:dbl, "Full Spectrum"=w234:T1)  [unwired: 2 out]
                            n115 = Multiply(x=1.2, y=w242) -> (x*y=w240:dbl)
                            n116 = Multiply(x=0.8, y=w242) -> (x*y=w237:dbl)
                            n117 = Less?(x=w233, y=w240) -> (x < y?=w239:bool)
                            n118 = Greater?(x=w233, y=w237) -> (0:w235:bool)
                            n119 = And(x=w239, y=w235) -> (x .and. y?=w238:bool)
                            n120 = case shown="True" w238 {
                              tunnel: [w276 w285] -> w245
                              tunnel: w234 -> [_ w280]
                              tunnel: w233 -> [_ w282]
                              frame False {
                                n121 = local read "Radial Load/ Rotor cracked"() -> (w276:T1)
                              }
                              frame True {
                                n122 = Unbundle(w280) -> ("order 0"=w279:dbl, "delta order"=w278:dbl, "magnitude"=w277:dbl[])
                                n123 = script code="order_max = -order;\nEixo_x = order:delta:order_max;\nEixo_xn=Eixo_x(1:round((end-1)/2));\nEixo_xp=Eixo_x(round(end/2+1):end);\nEixo_x = [Eixo_xn Eixo_xp];\nz = -2;\ni_min = find(Eixo_x >= (z-0.2));\ni_max = find(Eixo_x <= (z+0.2));\nYp= max(Mag(i_min(1):i_max(end)));\nY20 = Yp;\nz = 2;\ni_min = find(Eixo_x >= (z-0.2));\ni_max = find(Eixo_x <= (z+0.2));\nYp= max(Mag(i_min(1):i_max(end)));\nY21= Yp;\nY2=Y20+Y21;"("order"=w279, "delta"=w278, "Mag"=w277) -> ("Y2"=w281:dbl)  [unwired: 1 in, 1 out]
                                n124 = local read "Magcri2"() -> (w284:dbl)
                                n125 = Greater Or Equal?(x=w281, y=w284) -> (x >= y?=w283:bool)
                                n126 = case shown="True" w283 {
                                tunnel: w281 -> [_ w286]
                                frame False {
                                }
                                frame True {
                                "Magcri2" <- w286
                                }
                                }
                                n127 = case shown="True" w283 {
                                tunnel: w280 -> [_ w289]
                                tunnel: [w287 w289] -> w285
                                tunnel: w282 -> [_ w288]
                                frame False {
                                n128 = local read "Radial Load/ Rotor cracked"() -> (w287:T1)
                                }
                                frame True {
                                "Radial Load/ Rotor cracked" <- w289
                                "Freq [Hz]" <- w288
                                }
                                }
                              }
                            }
                            n129 = case shown="True" w235 {
                              tunnel: w234 -> [_ w253]
                              tunnel: w233 -> [_ w254]
                              tunnel: [FALSE w266] -> w232
                              tunnel: [w248 w255] -> w231
                              tunnel: [w247 w250] -> w230
                              frame False {
                                n130 = local read "owmax"() -> (w247:dbl)
                                n131 = local read "prmax"() -> (w248:dbl)
                              }
                              frame True {
                                n132 = call <vilib>:"Application Directory.vi"() -> ("Application Directory"=w258:path)
                                n133 = First Call?() -> (First Call?: T/F=w260:bool)
                                n134 = Unbundle(w253) -> ("order 0"=w265:dbl, "delta order"=w264:dbl, "magnitude"=w263:dbl[])
                                n135 = Path To String(path=w258) -> (string=w257:string)
                                n136 = Select(t=0.0, s=w260, f=1.0) -> (s? t:f=w259:dbl)
                                n137 = script code="switch i\ncase 0\naddfolder = '\\Fis files\\';\nfolder = strcat(cfolder,addfolder);\naddpath(folder)\nFis_ow = readfis('Fis_ow');\nFis_pr = readfis('Fis_pr');\n\n\n\norder_max = -order;\nEixo_x = order:delta:order_max;\nEixo_xn=Eixo_x(1:round((end-1)/2));\nEixo_xp=Eixo_x(round(end/2+1):end);\nEixo_x = [Eixo_xn Eixo_xp];\nk=1;\nfor z = [-2 -1 -0.5 0.5 1 2]\ni_min = find(Eixo_x >= (z-0.2));\ni_max = find(Eixo_x <= (z+0.2));\nYp(k) = max(Mag(i_min(1):i_max(end)));\nk = k+1;\nend\ndados_falha = Yp/max(Yp);\nfalha_ow = evalfis(dados_falha,Fis_ow);\nfalha_pr = evalfis(dados_falha,Fis_pr);\n\n\n\nFalha = [falha_ow falha_pr ];\nFalha(Falha>2) = 2;\nFalha(Falha<0) = 0;\now = 1-abs(1-Falha(1));\npr = 1-abs(1-Falha(2));\n\n\notherwise\n\norder_max = -order;\nEixo_x = order:delta:order_max;\nEixo_xn=Eixo_x(1:round((end-1)/2));\nEixo_xp=Eixo_x(round(end/2+1):end);\nEixo_x = [Eixo_xn Eixo_xp];\n\nk=1;\nfor z = [-2 -1 -0.5 0.5 1 2]\ni_min = find(Eixo_x >= (z-0.2));\ni_max = find(Eixo_x <= (z+0.2));\nYp(k) = max(Mag(i_min(1):i_max(end)));\nk = k+1;\nend\ndados_falha = Yp/max(Yp);\nfalha_ow = evalfis(dados_falha,Fis_ow);\nfalha_pr = evalfis(dados_falha,Fis_pr);\n\n\nFalha = [falha_ow falha_pr];\nFalha(Falha>2) = 2;\nFalha(Falha<0) = 0;\now = 1-abs(1-Falha(1));\npr = 1-abs(1-Falha(2));\n\nend"("order"=w265, "delta"=w264, "Mag"=w263, "i"=w259, "cfolder"=w257) -> ("??"=w268:errorcluster, "pr"=w256:dbl, "ow"=w251:dbl)  [unwired: 1 in]
                                "MATSCRIPT error 3" <- w268
                                n138 = local read "owmax"() -> (w250:dbl)
                                n139 = local read "prmax"() -> (w255:dbl)
                                n140 = Greater Or Equal?(x=w251, y=w250) -> (x >= y?=w252:bool)
                                n141 = Greater Or Equal?(x=w256, y=w255) -> (x >= y?=w269:bool)
                                n142 = case shown="True" w269 {
                                tunnel: w253 -> [_ w275]
                                tunnel: w254 -> [_ w274]
                                tunnel: w256 -> [_ w273]
                                frame False {
                                }
                                frame True {
                                "prmax" <- w273
                                "Partial Rub" <- w275
                                "Freq [Hz]" <- w274
                                }
                                }
                                n143 = case shown="True" w252 {
                                tunnel: w253 -> [_ w272]
                                tunnel: w254 -> [_ w271]
                                tunnel: w251 -> [_ w270]
                                frame False {
                                }
                                frame True {
                                "owmax" <- w270
                                "Oil Whirl" <- w272
                                "Freq [Hz]" <- w271
                                }
                                }
                                n144 = Unbundle By Name(w268) -> ("code"=w267:i32)
                                n145 = Not Equal To 0?(x=w267) -> (x != 0?=w266:bool)
                              }
                            }
                          }
                          "Unbalance" <- w214
                          "Freq [Hz]" <- w213
                          n146 = local write "Magcri2"(0.0 ("Magcrit2")) -> ()
                          n147 = local write "prmax"(0.0 ("subsync")) -> ()
                          n148 = local write "owmax"(0.0 ("subsync")) -> ()
                          n149 = First Call?() -> (First Call?: T/F=w223:bool)
                          n150 = call <vilib>:"Application Directory.vi"() -> ("Application Directory"=w220:path)
                          n151 = Select(t=0.0, s=w223, f=1.0) -> (s? t:f=w211:dbl)
                          n152 = Unbundle(w214) -> ("order 0"=w217:dbl, "delta order"=w216:dbl, "magnitude"=w215:dbl[])
                          n153 = Unbundle(w229) -> ("order 0"=w226:dbl, "delta order"=w225:dbl, "magnitude"=w224:dbl[])
                          n154 = Path To String(path=w220) -> (string=w212:string)
                          n155 = script code="switch i\ncase 0\naddfolder = '\\Fis files\\';\nfolder = strcat(cfolder,addfolder);\naddpath(folder)\nFis_rc = readfis('Fis_rc');\nFis_rl = readfis('Fis_rl');\norder_max = -order;\nEixo_x = order:delta:order_max;\nEixo_xn=Eixo_x(1:round((end-1)/2));\nEixo_xp=Eixo_x(round(end/2+1):end);\nEixo_x = [Eixo_xn Eixo_xp];\n\nk=1;\nfor z = [-2 -1 -0.5 0.5 1 2]\ni_min = find(Eixo_x >= (z-0.2));\ni_max = find(Eixo_x <= (z+0.2));\nYp(k) = max(Mag(i_min(1):i_max(end)));\nk = k+1;\nend\ndados_falha = Yp/max(Yp);\nfalha_rc = evalfis(dados_falha,Fis_rc);\nfalha_rl = evalfis(dados_falha,Fis_rl);\nFalha = [falha_rc falha_rl ];\nFalha(Falha>2) = 2;\nFalha(Falha<0) = 0;\nrc = 1-abs(1-Falha(1));\nrl = 1-abs(1-Falha(2));\n\n\notherwise\n\norder_max = -order;\nEixo_x = order:delta:order_max;\nEixo_xn=Eixo_x(1:round((end-1)/2));\nEixo_xp=Eixo_x(round(end/2+1):end);\nEixo_x = [Eixo_xn Eixo_xp];\ntam2=size(Eixo_x);\nk=1;\nfor z = [-2 -1 -0.5 0.5 1 2]\ni_min = find(Eixo_x >= (z-0.2));\ni_max = find(Eixo_x <= (z+0.2));\nYp(k) = max(Mag(i_min(1):i_max(end)));\nk = k+1;\nend\ndados_falha = Yp/max(Yp);\nfalha_rc = evalfis(dados_falha,Fis_rc);\nfalha_rl = evalfis(dados_falha,Fis_rl);\nFalha = [falha_rc falha_rl ];\nFalha(Falha>2) = 2;\nFalha(Falha<0) = 0;\nrc = 1-abs(1-Falha(1));\nrl = 1-abs(1-Falha(2));\nend"("order"=w226, "delta"=w225, "Mag"=w224, "i"=w211, "cfolder"=w212) -> ("??"=w228:errorcluster, "rc"=w208:dbl, "rl"=w207:dbl)  [unwired: 1 in]
                          "MATSCRIPT error 2" <- w228
                          n156 = script code="switch i\ncase 0\naddfolder = '\\Fis files\\';\nfolder = strcat(cfolder,addfolder);\naddpath(folder)\n\n\n\nFis_un = readfis('Fis_un');\norder_max = -order;\nEixo_x = order:delta:order_max;\nEixo_xn=Eixo_x(1:round((end-1)/2));\nEixo_xp=Eixo_x(round(end/2+1):end);\nEixo_x = [Eixo_xn Eixo_xp];\n\nk=1;\nfor z = [-2 -1 -0.5 0.5 1 2]\ni_min = find(Eixo_x >= (z-0.2));\ni_max = find(Eixo_x <= (z+0.2));\nYp(k) = max(Mag(i_min(1):i_max(end)));\nk = k+1;\nend\ndados_falha = Yp/max(Yp);\n\n\n\nfalha_un = evalfis(dados_falha,Fis_un);\nFalha = falha_un;\nFalha(Falha>2) = 2;\nFalha(Falha<0) = 0;\nun=1-abs(1-Falha);\n\n\notherwise\n\norder_max = -order;\nEixo_x = order:delta:order_max;\nEixo_xn=Eixo_x(1:round((end-1)/2));\nEixo_xp=Eixo_x(round(end/2+1):end);\nEixo_x = [Eixo_xn Eixo_xp];\ntam2=size(Eixo_x);\nk=1;\nfor z = [-2 -1 -0.5 0.5 1 2]\ni_min = find(Eixo_x >= (z-0.2));\ni_max = find(Eixo_x <= (z+0.2));\nYp(k) = max(Mag(i_min(1):i_max(end)));\nk = k+1;\nend\ndados_falha = Yp/max(Yp);\n\nfalha_un = evalfis(dados_falha,Fis_un);\nFalha = falha_un;\nFalha(Falha>2) = 2;\nFalha(Falha<0) = 0;\nun = 1-abs(1-Falha);\nend"("order"=w217, "delta"=w216, "Mag"=w215, "i"=w211, "cfolder"=w212) -> ("??"=w218:errorcluster, "un"=w209:dbl)  [unwired: 1 in]
                          "MATSCRIPT error" <- w218
                          n157 = Unbundle By Name(w218) -> ("code"=w219:i32)
                          n158 = Unbundle By Name(w228) -> ("code"=w227:i32)
                          n159 = Not Equal To 0?(x=w227) -> (x != 0?=w197:bool)
                          n160 = Not Equal To 0?(x=w219) -> (x != 0?=w196:bool)
                          n161 = Or(x=w196, y=w197) -> (x .or. y?=w198:bool)
                          n162 = Or(x=w198, y=w204) -> (x .or. y?=w210:bool)
                        }
                        frame True {
                          n163 = local read "Magcrit"() -> (w303:dbl)
                          n164 = Multiply(x=90.0, y=1.3) -> (x*y=w296:dbl)
                          n165 = Less?(x=w297, y=w296) -> (x < y?=w291:bool)
                          n166 = Greater?(x=w304, y=w303) -> (0:w292:bool)
                          n167 = And(x=w292, y=w291) -> (x .and. y?=w293:bool)
                          n168 = case shown="False" w293 {
                            tunnel: w307 -> [_ w310]
                            tunnel: [w308 w310] -> w306
                            tunnel: w304 -> [_ w309]
                            frame False {
                              n169 = local read "Freq crit"() -> (w308:dbl)
                            }
                            frame True {
                              "Magcrit" <- w309
                            }
                          }
                          "Freq crit" <- w306
                          "FreqFspec" <- w298
                          "deltaphase" <- w297
                        }
                      }
                      "Error Matlab Script" <- w182
                      "Unbalance" <- w181
                      "Rotor Crack" <- w180
                      "Radial Load" <- w179
                      "Partial Rub" <- w173
                      "Oil Whirl" <- w178
                      "Full Spectrum" <- w185
                    }
                  }
                }
              }
            }
            frame Error {
            }
          }
        }
        n170 = while {
          shift-right: [w390] -> _
          shift-left: waveform(dbl)[] [] ("appended array") -> [w389]
          shift-right: [w350] -> _
          shift-left: dbl[][] [] ("subarray") -> [w337]
          tunnel: w65 -> [w371]
          stop <- w368 stop-if-true
          # "num elementos na fila"
          # "Se tiver alguma coisa na fila,\nnem calculo nada, forçando \no desenfileiramento!\nAssim forço a \"limpeza da fila\""
          # "Colunas\nImpares = 1x\nPares      = 2x"
          # "A coluna 0 possui a frequencia"
          # "Colunas 7 e 8"
          # "Colunas 3 e 4"
          # "Colunas 5 e 6"
          # "Colunas 1 e 2"
          # "stop"
          n171 = Dequeue Element(queue=w371) -> (queue out=w370:refnum<queue>, element=w374:waveform(dbl)[], error out=w369:errorcluster)  [unwired: 2 in, 1 out]
          n172 = local read "even-angle references"() -> (w340:cluster{"r0":dbl, "dr":dbl, "Y":dbl[]}[])
          n173 = Get Queue Status(queue=w370, error in (no error)=w369) -> (error out=w368:errorcluster, # elements in queue=w373:i32)  [unwired: 1 in, 6 out]
          "error dequeue" <- w368
          "# elements in queue" <- w373
          n174 = feedback #1(dbl[] [] ("Y")) -> (w341:dbl[])
          n175 = Less?(x=w373, y=1) -> (x < y?=w367:bool)
          n176 = Not(x=w367) -> (.not. x?=→"> limit":bool)
          n177 = Index Array(array=w340, index=0) -> (element=w343:cluster{"r0":dbl, "dr":dbl, "Y":dbl[]})
          n178 = Unbundle By Name(w343) -> ("Y"=w345:dbl[])
          n179 = feedback-in #1(w345) -> ()
          n180 = Equal?(x=w341, y=w345) -> (x = y?=w346:bool[])
          n181 = Search 1D Array(1D array=w346, element=FALSE) -> (index of element=w348:i32)  [unwired: 1 in]
          n182 = Equal?(x=w348, y=-1) -> (x = y?=w339:bool)
          n183 = case shown="False" w339 {
            tunnel: [dbl[][] [] ("subarray") w392] -> w338
            tunnel: w337 -> [_ w392]
            frame False {
            }
            frame True {
            }
          }
          n184 = case shown="True" w367 {
            tunnel: w374 -> [w403 w422]
            tunnel: [w393 w421] -> w390
            tunnel: w389 -> [w407 w423]
            tunnel: [w411 w412] -> w350
            tunnel: w338 -> [w411 w416]
            frame False {
              # "Nessa etapa eu apenas armazeno\n os valores retornados pelo sensor."
              n185 = Index Array(array=w407, index=0 ("disabled index (col)")) -> (element=w402:waveform(dbl))
              n186 = Index Array(array=w407, index=1 ("disabled index (col)")) -> (element=w400:waveform(dbl))
              n187 = Index Array(array=w407, index=2 ("disabled index (col)")) -> (element=w398:waveform(dbl))
              n188 = Index Array(array=w403, index=0 ("disabled index (col)")) -> (element=w401:waveform(dbl))
              n189 = Index Array(array=w403, index=1 ("disabled index (col)")) -> (element=w399:waveform(dbl))
              n190 = Index Array(array=w403, index=2 ("disabled index (col)")) -> (element=w397:waveform(dbl))
              n191 = call-poly <vilib>:"Append Waveforms.vi"("waveform B"=w399, "waveform A"=w400) -> ("waveform out"=w395:waveform(dbl))  [unwired: 8 in, 1 out]
              n192 = call-poly <vilib>:"Append Waveforms.vi"("waveform B"=w401, "waveform A"=w402) -> ("waveform out"=w396:waveform(dbl))  [unwired: 8 in, 1 out]
              n193 = call-poly <vilib>:"Append Waveforms.vi"("waveform B"=w397, "waveform A"=w398) -> ("waveform out"=w394:waveform(dbl))  [unwired: 8 in, 1 out]
              n194 = Build Array(w396, w395, w394) -> (w393:waveform(dbl)[])
            }
            frame True {
              w448 = u16 0 items=["Rising", "Falling"] ("slope (Rising)")
              # "Para evitar tentar fazer \nconta com menos ciclos\ndo que o necessário \npara o bloco. \n30 ciclos para tentar calcular algo"
              # "Calcula a magnitude e phase dos sinais, \npara 1ª e 2ª ordem.\na. O bloco só retorna alguma coisa se tiver \nmais de 32 ciclos no sinal.\nb. Retorna apenas 1 valor de mag e phase, \npara uma das frequências no vetor de rotações.\n\nSendo assim, mesmo que o bloco MAG/PHASE \nseja executado, não é garantido que ele vai \nconseguir calcular um algum valor, por isso existe \na variável \"Data Available\" booleana na saida \""
              # "Separa as 3 wafeforms"
              # "Variáveis pra dizer \nse tem dados disponíveis"
              # "Vou criar um conjunto de dados onde calcula-se:\n\npos - função\n0 - frequência de rotação atual\n--------------------------------\n1 - Sensor X, 1x da freq. giro, mag\n2 - Sensor X, 2x da freq. giro, mag\n--------------------------------\n3 - Sensor Y, 1x da freq. giro, mag\n4 - Sensor Y, 2x da freq. giro, mag\n--------------------------------\n5 - Sensor X, 1x da freq. giro, fase\n6 - Sensor X, 2x da freq. giro, fase\n--------------------------------\n7 - Sensor Y, 1x da freq. giro, fase\n8 - Sensor Y, 2x da freq. giro, fase"
              n195 = local write "Threshold"("Threshold") -> ()
              n196 = call-poly <vilib>:"Index Waveform Array.vi"("index"=1, "waveform array"=w423) -> ("waveform"=w444:waveform(dbl))  [unwired: 8 in, 1 out]
              n197 = call-poly <vilib>:"Index Waveform Array.vi"("index"=2, "waveform array"=w423) -> ("waveform"=w450:waveform(dbl))  [unwired: 8 in, 1 out]
              n198 = call-poly <vilib>:"Index Waveform Array.vi"("index"=0, "waveform array"=w423) -> ("waveform"=w441:waveform(dbl))  [unwired: 8 in, 1 out]
              n199 = Unbundle By Name(w441) -> ("Y"=w440:dbl[])
              n200 = call <vilib>:"Waveform Min Max.vi"("waveform in"=w440) -> ("Y min"=w438:dbl, "Y max"=w443:dbl)  [unwired: 5 in, 4 out]
              n201 = Subtract(x=w443, y=w438) -> (x-y=w442:dbl)
              n202 = Divide(x=w442, y=2.0) -> (x/y=w436:dbl)
              n203 = Add(x=w438, y=w436) -> (x+y=w437:dbl)
              n204 = Unbundle By Name(w450) -> ("Y"=w451:dbl[])
              n205 = Unbundle By Name(w444) -> ("Y"=w452:dbl[])
              n206 = Subtract(x=w441, y=w437) -> (x-y=w439:waveform(dbl))
              n207 = call-poly <vilib>:"Mean.vi"("X"=w451) -> ("mean"=w457:dbl)  [unwired: 1 out]
              n208 = call-poly <vilib>:"Mean.vi"("X"=w452) -> ("mean"=w458:dbl)  [unwired: 1 out]
              n209 = Subtract(x=w450, y=w457) -> (x-y=w455:waveform(dbl))
              n210 = Subtract(x=w444, y=w458) -> (x-y=w456:waveform(dbl))
              n211 = call <vilib>:"OAT Analog Tacho Process (1 Tacho).vi"("analog tacho signal"=w439, "reset? (F)"=TRUE, "threshold (auto)"="Threshold", "slope (Rising)"=w448) -> ("speed profile"=w431:T12, "no tacho?"=→"no tacho?":bool, "error out"=w447:errorcluster)  [unwired: 7 in, 2 out]
              n212 = Unbundle By Name(w431) -> ("speed [RPM]"=w429:dbl[])
              n213 = Array Size(array=w429) -> (size(s)=w433:i32)
              "RPMs Calculados" <- w433
              n214 = Array Size(array=w429) -> (size(s)=w428:i32)
              n215 = Build Array(w456, w455) -> (w449:waveform(dbl)[])
              n216 = Decrement(x=w428) -> (x-1=w427:i32)
              n217 = Greater?(x=w433, y=30) -> (0:w430:bool)
              n218 = Index Array(array=w429, index=w427) -> (element=w426:dbl)
              n219 = case shown="True" w430 {
                tunnel: [_ w488] -> w413
                tunnel: w449 -> [_ w487]
                tunnel: [_ w486] -> w414
                tunnel: w447 -> [_ w485]
                tunnel: [FALSE ("Data Available") w481] -> w415
                tunnel: w431 -> [_ w482]
                frame False {
                }
                frame True {
                  n220 = local read "even-angle references"() -> (w480:cluster{"r0":dbl, "dr":dbl, "Y":dbl[]}[])
                  n221 = call "Mag_Phase_Calculator (SubVI).vi"("even-angle references"=w480, "error in (no error)"=w485, "view"=T8 {"dB on? (F)"=FALSE, "unwrap phase? (T)"=TRUE, "unit in degree? (T)"=TRUE}, "speed profile"=w482, "Array in"=w487) -> ("error out"=→"Mag/F":errorcluster, "Computed Mag/Phase"=w488:cluster{dbl, dbl, dbl, dbl}[], "RPS (Hz)"=w486:dbl, "Data Available"=w481:bool)  [unwired: 3 in]
                }
              }
              n222 = Divide(x=w426, y=60.0) -> (x/y=→"Rotation [rps]":dbl)
              n223 = case shown="True" w415 {
                tunnel: w416 -> [w461 w476]
                tunnel: [w461 w475] -> w412
                tunnel: w413 -> [_ w473]
                tunnel: w414 -> [_ w463]
                frame False {
                }
                frame True {
                  n224 = Index Array(array=w473, index=0) -> (element=w465:cluster{dbl, dbl, dbl, dbl})
                  n225 = Index Array(array=w473, index=1) -> (element=w466:cluster{dbl, dbl, dbl, dbl})
                  n226 = Unbundle(w465) -> (w462:dbl, w464:dbl, w472:dbl, w471:dbl)
                  n227 = Unbundle(w466) -> (w470:dbl, w469:dbl, w468:dbl, w467:dbl)
                  n228 = Build Array(w463, w462, w464, w472, w471, w470, w469, w468, w467) -> (w474:dbl[])
                  n229 = Insert Into Array(array=w476, new element=w474) -> (w475:dbl[][])  [unwired: 2 in]
                }
              }
              n230 = local read "Rotation [rps]"() -> (w419:dbl)
              n231 = local read "Actual Sample Rate (dt)"() -> (w420:dbl)
              n232 = call "Fifo (SubVI).vi"("duration"=200000.0, "y"=40.0, "Actual Sample Rate (dt)"=w420, "Rotation [RPS]"=w419, "Measurement in"=w422, "appended array"=w423) -> ("Array"=w421:waveform(dbl)[])  [unwired: 5 in]
              n233 = Wait Until Next ms Multiple(millisecond multiple=u32 100 ("milliseconds to wait")) -> ()  [unwired: 1 out]
            }
          }
          n234 = Index Array(array=w350, index (col)=0) -> (element=w353:dbl[])  [unwired: 1 in]
          n235 = Array Size(array=w353) -> (size(s)=w355:i32)
          n236 = Decrement(x=w355) -> (x-1=w352:i32)
          n237 = Index Array(array=w350, index (row) #1=w352, index (col) #1=0 ("index (col)"), index (row) #2=w352, index (col) #2=1 ("index (col)"), index (row) #3=w352, index (col) #3=3 ("index (col)"), index (col) #4=5 ("index (col)"), index (col) #5=7 ("index (col)")) -> (element #1=w351:dbl, element #2=w334:dbl, element #3=w333:dbl, element #4=w336:dbl[], element #5=w335:dbl[])  [unwired: 2 in]
          n238 = Add(x=i8 1, y="Order") -> (x+y=w386:i8)
          n239 = Add(x=i8 5, y="Order") -> (x+y=w383:i8)
          n240 = Add(x=i8 3, y="Order") -> (x+y=w377:i8)
          n241 = Add(x=i8 7, y="Order") -> (x+y=w380:i8)
          n242 = Max & Min(x=w334, y=w333) -> (max(x,y)=w361:dbl)  [unwired: 1 out]
          n243 = Greater?(x=w334, y=w333) -> (0:w332:bool)
          n244 = Index Array(array=w350, index (col)=0 ("index")) -> (element=w364:dbl[])  [unwired: 1 in]
          n245 = Index Array(array=w350, index (col)=w386) -> (element=w322:dbl[])  [unwired: 1 in]
          n246 = Index Array(array=w350, index (col)=w383) -> (element=w321:dbl[])  [unwired: 1 in]
          n247 = Index Array(array=w350, index (col)=w377) -> (element=w363:dbl[])  [unwired: 1 in]
          n248 = Index Array(array=w350, index (col)=w380) -> (element=w319:dbl[])  [unwired: 1 in]
          n249 = call "Unwrap (SubVI).vi"("phase in"=w336) -> ("phase out"=w331:dbl[])  [unwired: 9 in]
          n250 = call "Unwrap (SubVI).vi"("phase in"=w335) -> ("phase out"=w323:dbl[])  [unwired: 9 in]
          n251 = Array Max & Min(array=w331) -> (max value=w330:dbl, min value=w329:dbl)  [unwired: 2 out]
          n252 = Bundle("subarray"=w364, "subarray"=w322) -> (→"Magnitude":cluster{"subarray":dbl[], "subarray":dbl[]})  [unwired: 1 in]
          n253 = Bundle("subarray"=w364, "subarray"=w363) -> (→"Magnitude":cluster{"subarray":dbl[], "subarray":dbl[]})  [unwired: 1 in]
          n254 = call "Unwrap (SubVI).vi"("phase in"=w319) -> ("phase out"=w318:dbl[])  [unwired: 9 in]
          n255 = Bundle("subarray"=w364, "phase out"=w318) -> (→"Phase":cluster{"subarray":dbl[], "phase out":dbl[]})  [unwired: 1 in]
          n256 = call "Unwrap (SubVI).vi"("phase in"=w321) -> ("phase out"=w320:dbl[])  [unwired: 9 in]
          n257 = Bundle("subarray"=w364, "phase out"=w320) -> (→"Phase":cluster{"subarray":dbl[], "phase out":dbl[]})  [unwired: 1 in]
          n258 = Subtract(x=w330, y=w329) -> (x-y=w328:dbl)
          n259 = Array Max & Min(array=w323) -> (max value=w326:dbl, min value=w327:dbl)  [unwired: 2 out]
          n260 = Subtract(x=w326, y=w327) -> (x-y=w325:dbl)
          n261 = Select(t=w328, s=w332, f=w325) -> (s? t:f=w324:dbl)
          n262 = Build Array(w351, w361, w324) -> (→"RotMagdeltaphase":dbl[])
        }
        n263 = TDMS Close(8:w55, 11:w56) -> (0:w70:errorcluster)  [unwired: 1 out]
        n264 = call <vilib>:"DAQmx Stop Task.vi"("task/channels in"=w92, "error in"=w91) -> ("task out"=w89:refnum<k21>, "error out"=w90:errorcluster)  [unwired: 12 in]
        n265 = Release Queue(queue=w78, error in (no error)=w77) -> (error out=w51:errorcluster)  [unwired: 3 out]
        n266 = Release Queue(queue=w74, error in (no error)=w72) -> (error out=w73:errorcluster)  [unwired: 1 in, 2 out]
        n267 = Release Queue(queue=w86, error in (no error)=w79) -> (error out=w52:errorcluster)  [unwired: 3 out]
        n268 = call <vilib>:"DAQmx Clear Task.vi"("task in"=w89, "error in"=w90) -> ("error out"=w66:errorcluster)  [unwired: 13 in]
        n269 = Merge Errors(w66, w52, w51, w73, w70) -> (w62:errorcluster)
        n270 = call <vilib>:"Simple Error Handler.vi"("type of dialog (OK msg:1)"=w88, "error in (no error)"=w62) -> ()  [unwired: 8 out]
        n271 = property on="Simulation" class="Bool (strict)"("DisabledEnum"=T6."Disabled and Grayed Out" ("Disabled")) -> ()  [unwired: 2 in, 2 out]
      }
    }
    n272 = Wait Until Next ms Multiple(millisecond multiple=u32 50) -> ()  [unwired: 1 out]
    "State" <- w9
  }
